vi "Is Configuration Valid.vi"(8 "error in":errorcluster, 11 "Lv Proj Document Type:TAF Proj":refnum<class "TAF Proj.lvclass">) -> (0 "error out":errorcluster, 1 "Details":string, 2 "Valid?":bool, 3 "Lv Proj Document Type:TAF Proj":refnum<class "TAF Proj.lvclass">)   [LabVIEW 2021, in "TAF Proj Document Type.lvlib" / "TAF Proj.lvclass"]
uses:
  <vilib>/Wovalab/AntiDoc/Document Type/Add-ons/LabVIEW TAF Project/TAF Proj/TAF Proj.lvclass
  C:/Program Files (x86)/National Instruments/LabVIEW 2021/vi.lib/Wovalab/AntiDoc/Document Type/Document/Document Type.lvclass
  <vilib>/Wovalab/AntiDoc/Document Type/Add-ons/LabVIEW TAF Project/TAF Proj Config/TAF Proj Config.lvclass
  <vilib>/Wovalab/AntiDoc/Document Type/Document/Document Type.lvclass/Document Type.ctl
  <vilib>/Wovalab/AntiDoc/Document Type/Add-ons/LabVIEW TAF Project/TAF Proj Config/TAF Proj Config.lvclass/TAF Proj Config.ctl
  <vilib>/Wovalab/AntiDoc/Document Type/Document/Read Config.vi
  <vilib>/Wovalab/AntiDoc/Document Type/Add-ons/LabVIEW TAF Project/TAF Proj Config/Read Project Path.vi
  <vilib>/Wovalab/AntiDoc/Document Type/Config/Config.lvclass
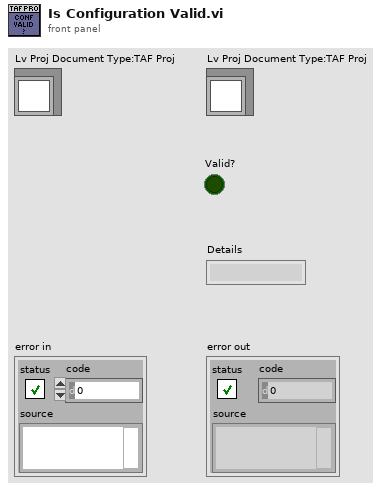
[diagram p1: front panel]
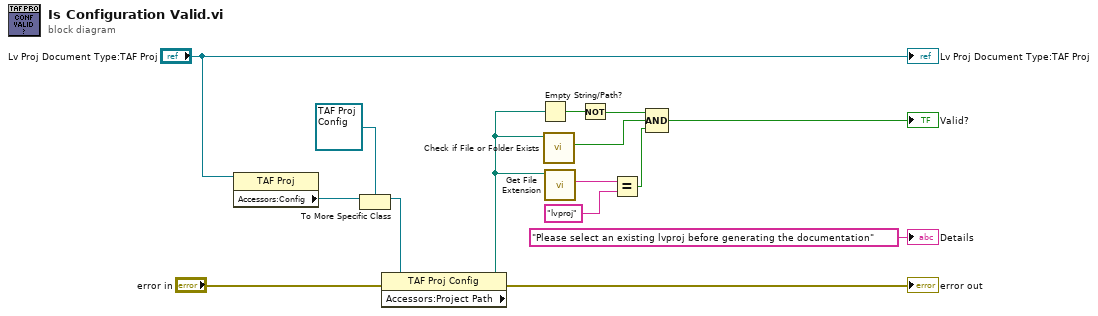
[diagram p0: block diagram]
diagram:
  n1 = property class="TAF Proj"(reference="Lv Proj Document Type:TAF Proj") -> ("Accessors:Config"=w4:refnum<class "Config.lvclass">)  [unwired: 1 in, 2 out]
  n2 = To More Specific Class(target class=refnum<class "TAF Proj Config.lvclass"> refnum ("Lv Proj Document Type.lvlib:Config"), reference=w4) -> (specific class reference=w1:refnum<class "TAF Proj Config.lvclass">)  [unwired: 1 in, 1 out]
  n3 = property class="TAF Proj Config"(reference=w1, error in="error in") -> (error out=→"error out":errorcluster, "Accessors:Project Path"=w5:path)  [unwired: 1 out]
  n4 = Empty String/Path?(string/path=w5) -> (empty?=w13:bool)
  n5 = call <vilib>:"Check if File or Folder Exists.vi"("path"=w5) -> ("file or folder exists?"=w9:bool)  [unwired: 8 in, 2 out]
  n6 = call <vilib>:"Get File Extension.vi"("file"=w5) -> ("lowercase file extension"=w12:string)  [unwired: 6 in, 4 out]
  n7 = Not(x=w13) -> (.not. x?=w10:bool)
  n8 = Equal?(x=w12, y="lvproj") -> (x = y?=w8:bool)
  n9 = Compound Arithmetic op=AND(w10, w9, w8) -> (→"Valid?":bool)
  "Lv Proj Document Type:TAF Proj" <- "Lv Proj Document Type:TAF Proj"
  "Details" <- "Please select an existing lvproj before generating the documentation" ("Details")
